vi "IntakeSetDemands.vi"(8 "turntableDemand":dbl) -> ()   [LabVIEW 2020]
doc: "sets values to the intake global variables\n\nInputs\n--intakeUpper Demand--Double\n--intakeLowerDemand--Double\n--turntableDemand--Double"
uses:
  IntakeGlobal.vi
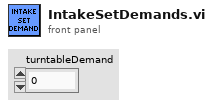
[diagram p1: front panel]
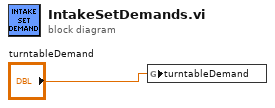
[diagram p0: block diagram]
diagram:
  n1 = global write "IntakeGlobal.vi" "turntableDemand"("turntableDemand") -> ()
